vi "Add Sibling.vi"(8 "error in (no error)":errorcluster, 10 "Sibling":refnum<data-value>, 11 "NodeRef In":refnum<data-value>) -> (0 "error out":errorcluster, 3 "NodeRef":refnum<data-value>)   [LabVIEW 2020, in "PicoG-ParserLexer.lvlib" / "Node.lvclass"]
doc: "Adds a new sibling to the end of the current sibling list. If nodes are have the same parent (They are already siblings) then no action is taken. New sibling must not have a parent assigned already.\n\n<b>Error Codes:</b>\n<b>14</b>: New sibling already has a parent assigned. To move a node around the tree it must be removed from its parent with RemoveChild first.\n<b>1556</b>: One of the nodes is not instantiated; call Ctor for the instance first."
uses:
  Node.lvclass
  <vilib>/ErrorRing/Error Ring.xnode
  <vilib>/Utility/error.llb/Error Cluster From Error Code.vi
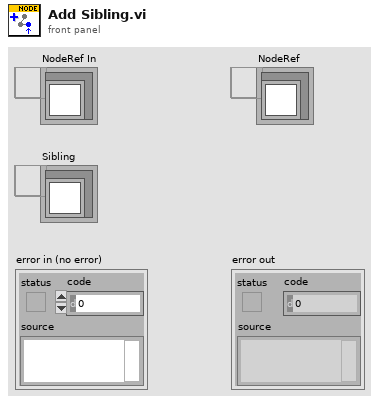
[diagram p1: front panel]
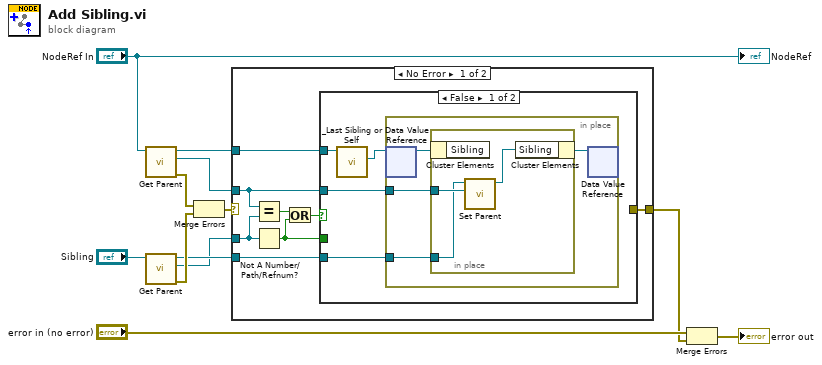
[diagram p0: block diagram]
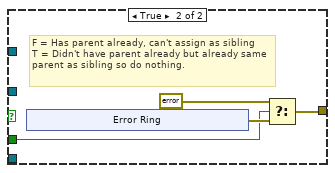
[diagram p2: hidden frame]
diagram:
  n1 = call "Get Parent.vi"("NodeRef In"="NodeRef In") -> ("error out"=w7:errorcluster, "Parent"=w6:refnum<data-value>, "NodeRef"=w4:refnum<data-value>)  [unwired: 8 in]
  n2 = call "Get Parent.vi"("NodeRef In"="Sibling") -> ("error out"=w12:errorcluster, "Parent"=w2:refnum<data-value>, "NodeRef"=w8:refnum<data-value>)  [unwired: 8 in]
  n3 = Merge Errors(w7, w12) -> (w3:errorcluster)
  n4 = case shown="No Error" w3 {
    selector: w3 -> [_ w40]
    tunnel: w8 -> [w20 _]
    tunnel: w6 -> [w13 _]
    tunnel: [w14 w40] -> w5
    tunnel: w4 -> [w19 _]
    tunnel: w2 -> [w18 _]
    frame No Error {
      n5 = Equal?(x=w13, y=w18) -> (x = y?=w17:bool)
      n6 = Not A Number/Path/Refnum?(number/path/refnum=w18) -> (NaN/Path/Refnum?=w15:bool)
      n7 = Or(x=w17, y=w15) -> (x .or. y?=w16:bool)
      n8 = case shown="False" w16 {
        tunnel: w20 -> [w24 _]
        tunnel: w19 -> [w22 _]
        tunnel: w15 -> [_ w34]
        tunnel: [_ w32] -> w14
        tunnel: w13 -> [w23 _]
        frame False {
          n9 = call "_Last Sibling or Self.vi"("NodeRef In"=w22) -> ("Last Sibling or Self"=w21:refnum<data-value>)  [unwired: 8 in, 2 out]
          n10 = in-place {
            in-place-border: w24 -> [w27]
            in-place-border: w23 -> [w26]
            n11 = in-place-dvr #1(w21) -> (w28:refnum<class "Node.lvclass">)  [unwired: 1 out]
            n12 = in-place {
              in-place-border: w27 -> [w30]
              in-place-border: w26 -> [w31]
              n13 = in-place-cluster #2(w28) -> ()  [unwired: 1 out]
              n14 = call "Set Parent.vi"("Parent"=w31, "NodeRef In"=w30) -> ("NodeRef"=w29:refnum<data-value>)  [unwired: 8 in, 1 out]
              n15 = in-place-cluster #2("Sibling"=w29) -> (w25:refnum<class "Node.lvclass">)
            }
            n16 = in-place-dvr #1(w25) -> ()  [unwired: 2 out]
          }
        }
        frame True {
          # "F = Has parent already, can't assign as sibling\nT = Didn't have parent already but already same parent as sibling so do nothing."
          n17 = xnode "Error Ring"() -> ("error out"=w35:errorcluster)
          n18 = Select(t=errorcluster {"status"=FALSE, "code"=0, "source"=""} ("f"), s=w34, f=w35) -> (s? t:f=w32:errorcluster)
        }
      }
    }
    frame Error {
    }
  }
  n19 = Merge Errors("error in (no error)", w5) -> (→"error out":errorcluster)
  "NodeRef" <- "NodeRef In"
